vi "GetParticleResultNames.vi"(7 "ProjectName":string="Prj", 10 "data":T2={"Clamp Settings"={"Contrast"=40, "Filter width"=4, "Steepness"=2, "Subsampling Ratio"=5, "Show Search Area"=TRUE, "Show Search Lines"=TRUE, "Show Edges Found"=TRUE, "Show Result"=TRUE}, "ROI Descriptor"={"Global Rectangle"=[], "Contours"=[]}, "Process"=0}, 11 "ROI_Name":string="ROI1") -> (3 "ResultNames":string[](array[string]))   [LabVIEW 2015]
uses:
  Controls/Clamp/Analysis_Clamp_Parameter.ctl
  Controls/Clamp/Analysis_Clamp_Result.ctl
panel:
  in  "Analysis_Clamp_Result":T1 {"Edge Point"."Y" format="%.2f"; "Edge Point"."X" format="%.2f"}
  out "error out":errorcluster
  in  "error in (no error)":errorcluster
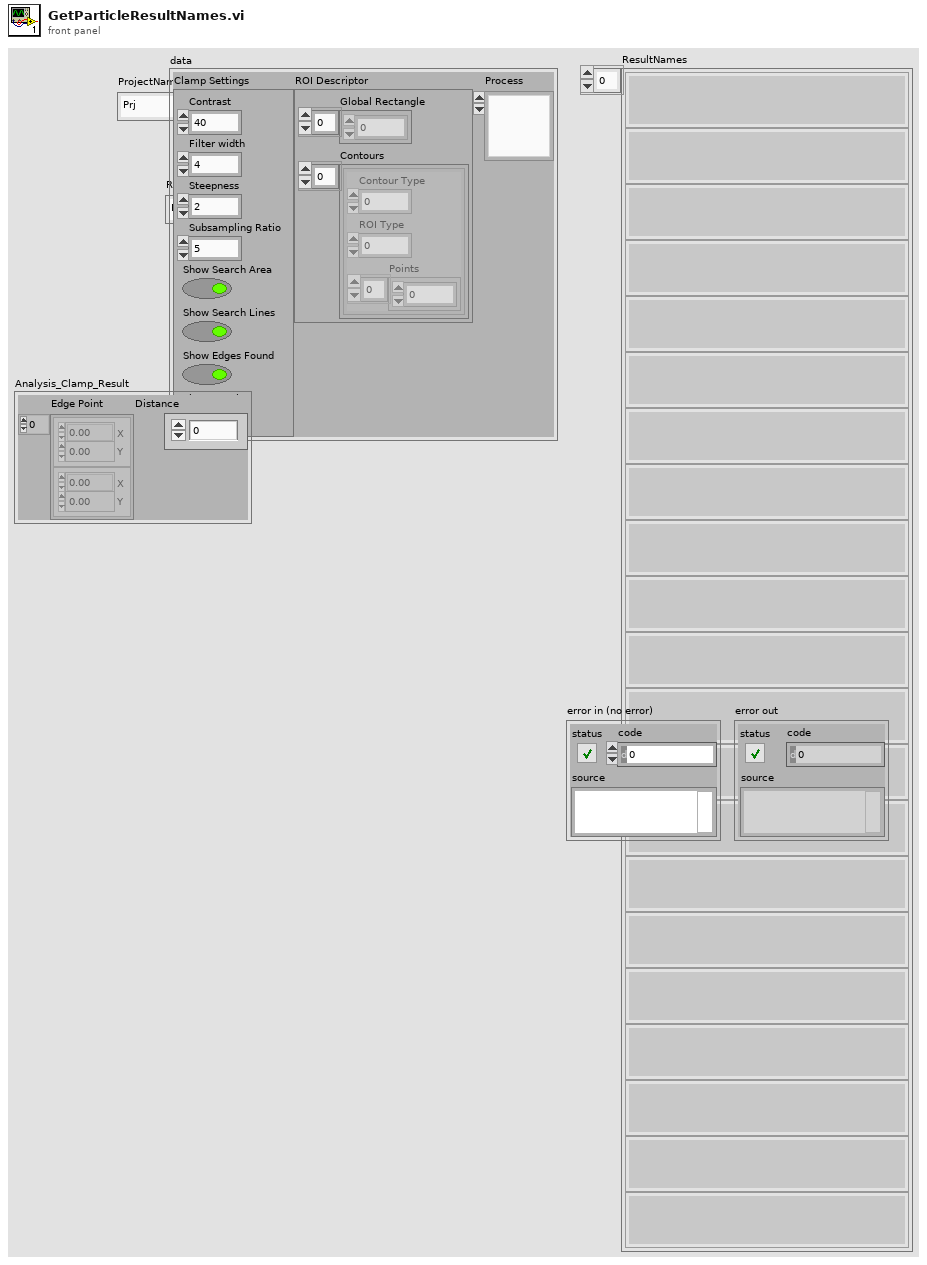
[diagram p1: front panel]
types:
  T1 = typedef "Analysis_Clamp_Result.ctl" = cluster{"Edge Point":cluster{"X":sgl, "Y":sgl}[], "Distance":sgl}
  T2 = typedef "Analysis_Clamp_Parameter.ctl" = cluster{"Clamp Settings":cluster{"Contrast":i32, "Filter width":i32, "Steepness":i32, "Subsampling Ratio":u32, "Show Search Area":bool, "Show Search Lines":bool, "Show Edges Found":bool, "Show Result":bool}, "ROI Descriptor":cluster{"Global Rectangle":i32[], "Contours":cluster{"Contour Type":u32, "ROI Type":u32, "Points":i32[]}[]}, "Process":u16}
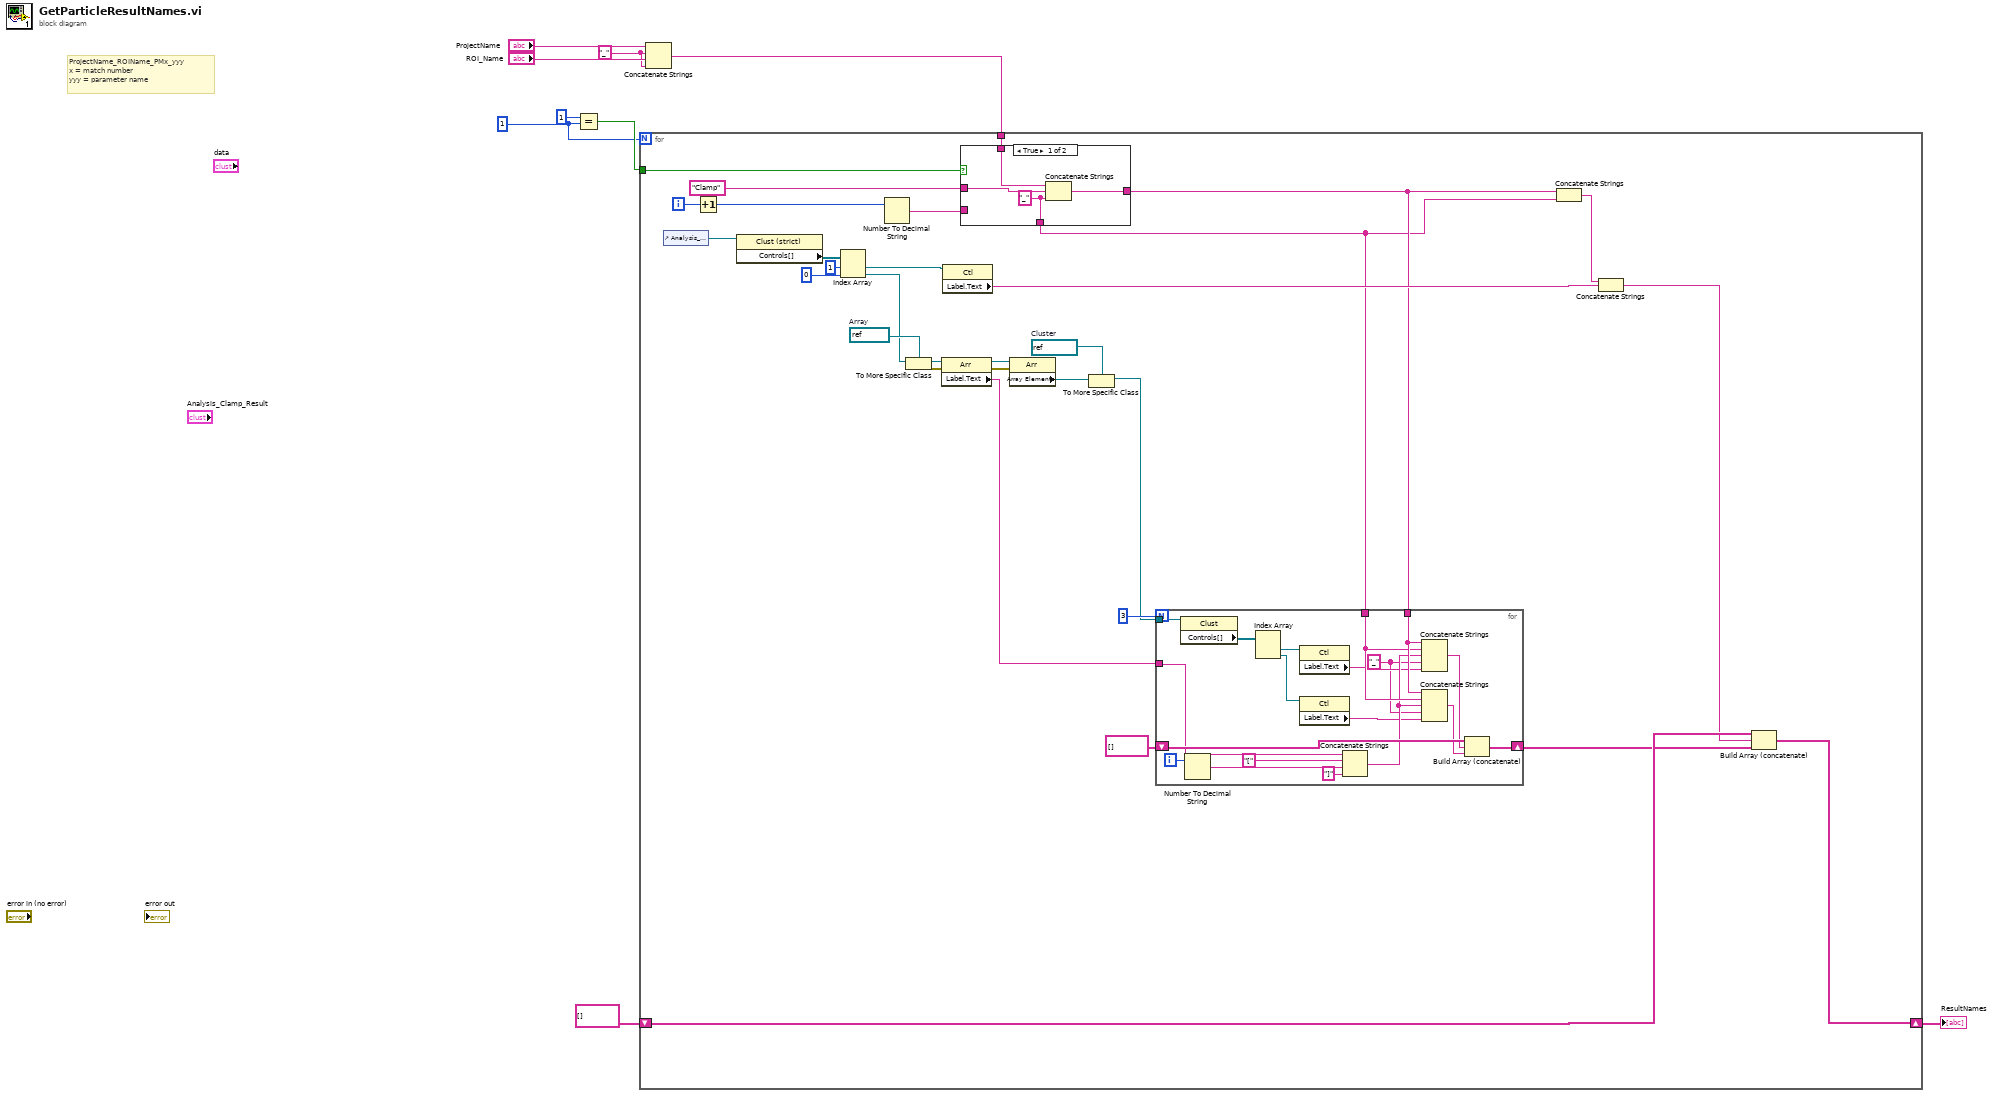
[diagram p0: block diagram]
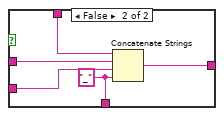
[diagram p2: hidden frame]
diagram:
  w1 = 1
  w6 = "_" ("string")
  # "ProjectName_ROIName_PMx_yyy\nx = match number\nyyy = parameter name"
  n1 = Equal?(x=1, y=w1) -> (x = y?=w2:bool)
  n2 = Concatenate Strings("ProjectName", w6, "ROI_Name", w6) -> (w5:string)
  n3 = for {
    N: w1 -> [_]
    tunnel: w5 -> [w38]
    shift-right: [w30] -> w3
    shift-left: string[] [] -> [w34]
    tunnel: w2 -> [w39]
    i -> [w35]
    w14 = refnum<vi> refnum  # Cluster
    w27 = refnum<vi> refnum  # Array
    n4 = control-ref of="Analysis_Clamp_Result"() -> (w28:refnum<vi>)
    n5 = Increment(x=w35) -> (x+1=w40:i32)
    n6 = property class="Clust (strict)"(reference=w28) -> ("Controls[]"=w32:refnum<vi>[])  [unwired: 1 in, 2 out]
    n7 = Index Array(array=w32, index #1=1 ("index"), index #2=0) -> (element #1=w21:refnum<vi>, element #2=w26:refnum<vi>)
    n8 = Number To Decimal String(number=w40) -> (decimal integer string=w37:string)  [unwired: 1 in]
    n9 = To More Specific Class(target class=w27, reference=w26) -> (specific class reference=w25:refnum<vi>, error out=w24:errorcluster)  [unwired: 1 in]
    n10 = property class="Arr"(reference=w25, error in=w24) -> (reference out=w23:refnum<vi>, error out=w22:errorcluster, "Label.Text"=w11:string)
    n11 = property class="Ctl"(reference=w21) -> ("Label.Text"=w20:string)  [unwired: 1 in, 2 out]
    n12 = case shown="True" w39 {
      tunnel: w38 -> [w63 w68]
      tunnel: w37 -> [_ w66]
      tunnel: [w62 w67] -> w17
      tunnel: "Clamp" ("string") -> [w61 w65]
      tunnel: [w60 w64] -> w16
      frame True {
        w60 = "_" ("string")
        n13 = Concatenate Strings(w63, w61, w60) -> (w62:string)
      }
      frame False {
        w64 = "_" ("string")
        n14 = Concatenate Strings(w68, w65, w66, w64) -> (w67:string)
      }
    }
    n15 = property class="Arr"(reference=w23, error in=w22) -> ("Array Element"=w15:refnum<vi>)  [unwired: 2 out]
    n16 = To More Specific Class(target class=w14, reference=w15) -> (specific class reference=w13:refnum<vi>)  [unwired: 1 in, 1 out]
    n17 = for {
      N: 3 -> [_]
      tunnel: w11 -> [w51]
      tunnel: w13 -> [w59]
      tunnel: w17 -> [w58]
      tunnel: w16 -> [w57]
      shift-right: [w53] -> w10
      shift-left: string[] [] -> [w56]
      i -> [w52]
      w45 = "_" ("string")
      n18 = property class="Clust"(reference=w59) -> ("Controls[]"=w44:refnum<vi>[])  [unwired: 1 in, 2 out]
      n19 = Number To Decimal String(number=w52) -> (decimal integer string=w49:string)  [unwired: 1 in]
      n20 = Index Array(array=w44) -> (element #1=w43:refnum<vi>, element #2=w41:refnum<vi>)  [unwired: 2 in]
      n21 = property class="Ctl"(reference=w43) -> ("Label.Text"=w46:string)  [unwired: 1 in, 2 out]
      n22 = property class="Ctl"(reference=w41) -> ("Label.Text"=w42:string)  [unwired: 1 in, 2 out]
      n23 = Concatenate Strings(w51, "[" ("string"), w49, "]" ("string")) -> (w47:string)
      n24 = Concatenate Strings(w58, w57, w47, w45, w46) -> (w55:string)
      n25 = Concatenate Strings(w58, w57, w47, w45, w42) -> (w54:string)
      n26 = Build Array (concatenate)(w56, w55, w54) -> (w53:string[])
    }
    n27 = Concatenate Strings(w17, w16) -> (w33:string)
    n28 = Concatenate Strings(w33, w20) -> (w19:string)
    n29 = Build Array (concatenate)(w34, w19, w10) -> (w30:string[])
  }
  "ResultNames" <- w3
